vi "字符串截取，并输出波形数组.vi"(11 "read buffer":string) -> (1 "字节描述数据的长度":i32, 2 "数据长度":i32, 3 "数组":u8[](array[numeric]))   [LabVIEW 2018]
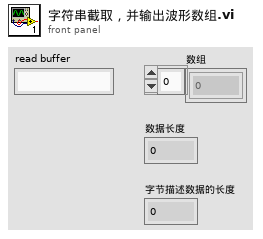
[diagram p1: front panel]
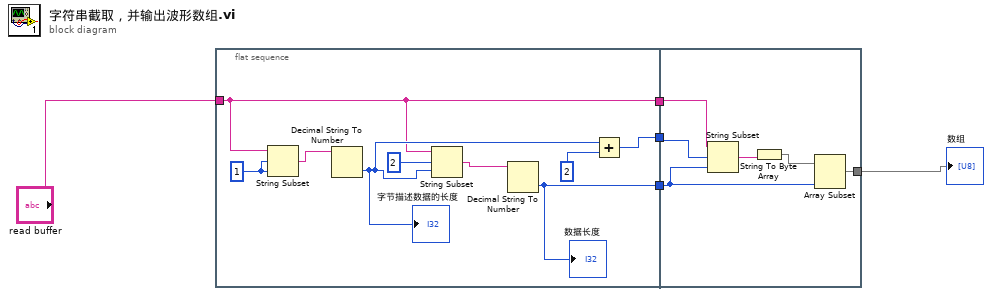
[diagram p0: block diagram]
diagram:
  n1 = flat-sequence {
    tunnel: [w6] -> w5
    tunnel: [w9] -> w4
    tunnel: [w8] -> w3
    tunnel: "read buffer" -> [w6]
    tunnel: w5 -> [w19]
    tunnel: w4 -> [w20]
    tunnel: w3 -> [w16]
    tunnel: [w15] -> w2
    frame #0 {
      w11 = 1 ("偏移量(0)")
      n2 = String Subset(string=w6, offset (0)=w11, length (rest)=w11) -> (substring=w13:string)
      n3 = Decimal String To Number(string=w13) -> (number=w7:i32)  [unwired: 2 in, 1 out]
      "字节描述数据的长度" <- w7
      n4 = String Subset(string=w6, offset (0)=2 ("偏移量(0)"), length (rest)=w7) -> (substring=w14:string)
      n5 = Decimal String To Number(string=w14) -> (number=w8:i32)  [unwired: 2 in, 1 out]
      "数据长度" <- w8
      n6 = Add(x=w7, y=2) -> (x+y=w9:i32)
    }
    frame #1 {
      n7 = String Subset(string=w19, offset (0)=w20, length (rest)=w16) -> (substring=w18:string)
      n8 = String To Byte Array(string=w18) -> (unsigned byte array=w17:u8[])
      n9 = Array Subset(array=w17, length=w16) -> (w15:u8[])  [unwired: 1 in]
    }
  }
  "数组" <- w2
